vi "Fdx Create Session (Generic-Port).vi"(8 "error in (no error)":errorcluster, 10 "port":u32, 11 "board":u32) -> (0 "error out":errorcluster, 2 "InstrumentHandle_port out":u32, 3 "InstrumentHandle_board out":u32, 4 "Duplicated":bool)   [LabVIEW 2020, in "AIM664LV.lvlib"]
uses:
  AIM664LV.lvlib
  _controls/hwEntry_actions.ctl
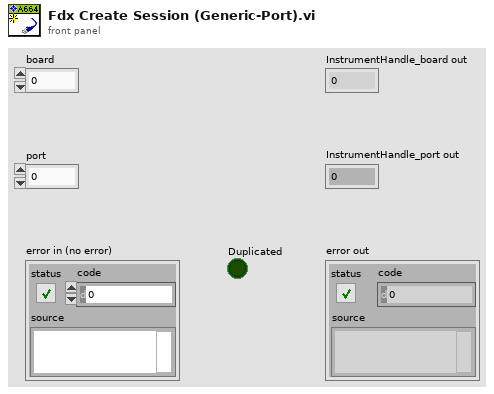
[diagram p1: front panel]
types:
  T1 = typedef "AIM664LV.lvlib/hwEntry_actions.ctl" = enum16{"Init Port", "Init Board", "Relase Port", "Release Board"}
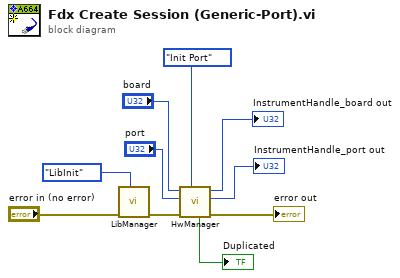
[diagram p0: block diagram]
diagram:
  n1 = call "LibManager.vi"("action"=enum16{"LibInit", "LibExit"}."LibInit", "error in (no error)"="error in (no error)") -> ("error out"=w8:errorcluster)  [unwired: 7 in, 2 out]
  n2 = call "HwManager.vi"("action (Init)"=hwEntry_actions."Init Port" ("action"), "error in (no error)"=w8, "port"="port", "board"="board") -> ("error out"=→"error out":errorcluster, "InstrumentHandle_port out"=→"InstrumentHandle_port out":u32, "InstrumentHandle_board out"=→"InstrumentHandle_board out":u32, "Duplicated"=→"Duplicated":bool)  [unwired: 3 in, 1 out]
